vi "Close.vi"(8 "error in (no error)":errorcluster, 11 "uService Template in":refnum<class "New uService Template.lvclass">) -> (0 "error out":errorcluster, 3 "uService Template out":refnum<class "New uService Template.lvclass">)   [LabVIEW 2021, in "New uService Template.lvlib" / "New uService Template.lvclass"]
uses:
  New uService Template.lvclass
  TALOS/TALOS_PPL.lvlibp/Father of all uServices/Father of all uServices/Father of all uServices.lvclass
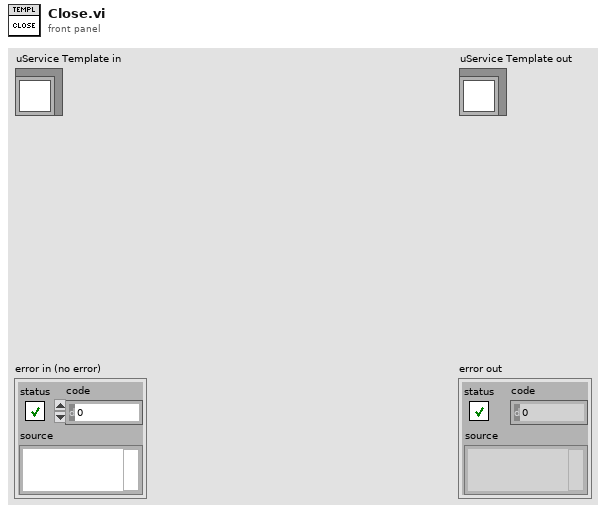
[diagram p1: front panel]
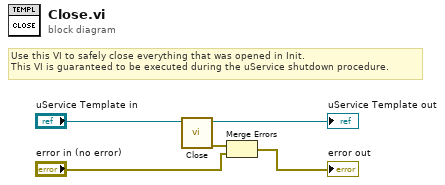
[diagram p0: block diagram]
diagram:
  # "Use this VI to safely close everything that was opened in Init.\nThis VI is guaranteed to be executed during the uService shutdown procedure."
  n1 = call-parent "Close.vi"("uService Template in"="uService Template in") -> ("error out"=w5:errorcluster, "uService Template out"=→"uService Template out":refnum<class "New uService Template.lvclass">)  [unwired: 9 in]
  n2 = Merge Errors(w5, "error in (no error)") -> (→"error out":errorcluster)
